vi "Set Default (DBL).vi"(8 "error in (no error)":errorcluster, 10 "Default":dbl, 11 "Channel in":refnum<class "Channel.lvclass">) -> (0 "error out":errorcluster, 3 "Channel out":refnum<class "Channel.lvclass">)   [LabVIEW 2020, in "VolatusConfig.lvlib" / "Channel.lvclass"]
uses:
  Channel.lvclass
  Channel.lvclass/Channel.ctl
  VolatusConfigElement/VolatusConfigElement.lvclass
  lv-cdm/CDM-Config/Config Element/Config Element.lvclass
  lv-cdm/CDM-Config/Value Type.ctl
  lv-cdm/CDM-Config/CDM-Config.lvlib
  C:/dev/lv20CE/relink/lv-volatus/VolatusConfig/VolatusConfigElement/VolatusConfigElement.lvclass
  C:/dev/lv20CE/relink/lv-volatus/VolatusConfig/Channel/Channel.lvclass
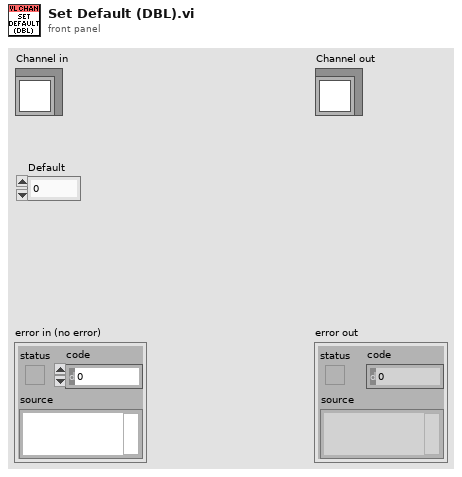
[diagram p1: front panel]
types:
  T1 = typedef "CDM-Config.lvlib/Value Type.ctl" = enum16{"String", "Number", "Bool", "Object", "Array"}
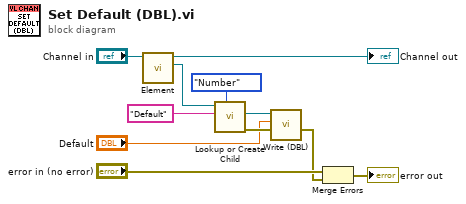
[diagram p0: block diagram]
diagram:
  n1 = call "Element.vi"("VolatusConfigElement in"="Channel in") -> ("Element"=w8:refnum<class "Config Element.lvclass">, "VolatusConfigElement out"=→"Channel out":refnum<class "Channel.lvclass">)  [unwired: 9 in]
  n2 = call "Lookup or Create Child.vi"("Value Type (String)"=Value_Type."Number", "Name"="Default", "Config Element in"=w8) -> ("error out"=w5:errorcluster, "Child"=w4:refnum<class "Config Element.lvclass">)  [unwired: 5 in, 2 out]
  n3 = call "Write (DBL).vi"("error in (no error)"=w5, "DBL Value"="Default", "Config Element in"=w4) -> ("error out"=w1:errorcluster)  [unwired: 7 in, 1 out]
  n4 = Merge Errors("error in (no error)", w1) -> (→"error out":errorcluster)
